vi "写入填充.vi"(8 "error in (no error)":errorcluster caption="错误输入（无错误）", 10 "填充":bool, 11 "图形输入":refnum<class "图形.lvclass">) -> (0 "error out":errorcluster caption="错误输出", 3 "图形输出":refnum<class "图形.lvclass">)   [LabVIEW 2011, in "图形.lvclass"]
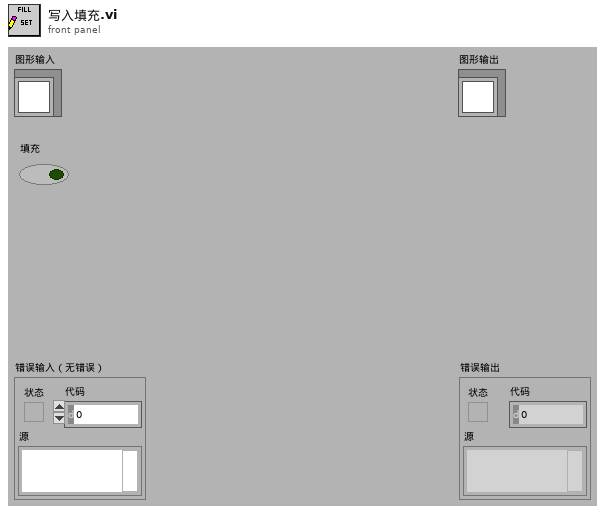
[diagram p1: front panel]
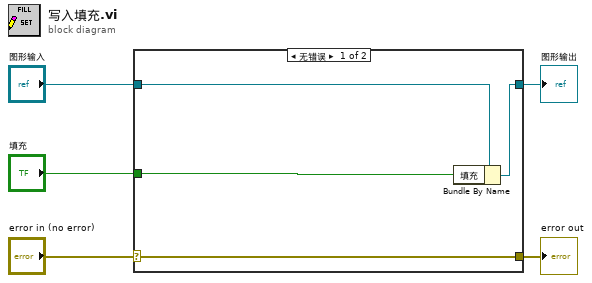
[diagram p0: block diagram]
diagram:
  n1 = case shown="无错误" "error in (no error)" {
    selector: "error in (no error)" -> [w9 w10]
    tunnel: [w9 w10] -> w4
    tunnel: [w7 w11] -> w2
    tunnel: "图形输入" -> [w8 w11]
    tunnel: "填充" -> [w6 _]
    frame No Error {
      n2 = Bundle By Name(cluster=w8, "填充"=w6) -> (w7:refnum<class "图形.lvclass">)
    }
    frame Error {
    }
  }
  "error out" <- w4
  "图形输出" <- w2
